vi "String Label.vi"(9 "i":i32, 10 "Label in":string) -> (2 "Label+i out":string)   [LabVIEW 2019, in "Control Experiment.lvclass"]
uses:
  Control Experiment.lvclass
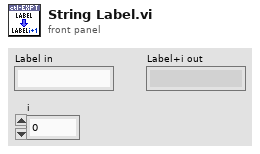
[diagram p1: front panel]
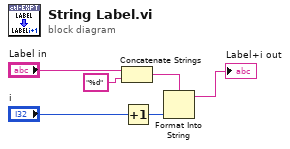
[diagram p0: block diagram]
diagram:
  n1 = Concatenate Strings("Label in", "%d" ("wavenames")) -> (w4:string)
  n2 = Increment(x="i") -> (x+1=w3:i32)
  n3 = Format Into String(format string=w4, w3) -> (resulting string=→"Label+i out":string)  [unwired: 2 in, 1 out]
